vi "Startup_Main.vi"(11 "Message Steps Ref":refnum<vi>) -> (1 "path":path)   [LabVIEW 2016]
doc: "Follow the below steps:\n1) Run the VI\n2) 1st State is \"Wait For Start Acquisition\"\nSelect the \"StartAcquisition\" from States-Enum and Press Send External Trigger button\n3) 2nd State is \"Read Configuration\"\nSelect the \"CheckConfigChanged\" from States-Enum and Press Send External Trigger button\n4) 3rd State is \"Create Channels\"\nThis will Popup a message and automatically goes to next state\n5) 4th State is \"Start Task\"\nThis will Popup a message and automatically goes to next state\n6) 5th State is \"Acquire Data\"\nThe logic will wait here until the \"StopAcq\" or \"Shutdown\" triggers are received\n7) Select the \"StopAcq\" from States-Enum and Press Send External Trigger button\nThis will Popup a message and automatically goes to first state\n\nNote: \nAny state where the logic is waiting, you can Select the \"StopAcq\" from States-Enum and Press Send External Trigger button\n- This will popup a message and automatically goes to first state\nAny state where the logic is waiting, you can Select the \"Shutdown\" from States-Enum and Press Send External Trigger button\n- This will execute the Shutdown state and terminate the program\nBy Manish Soni"
uses:
  Startup_States.ctl
panel:
  out "path 2":path
  out "Paths":T1
  out "String":string
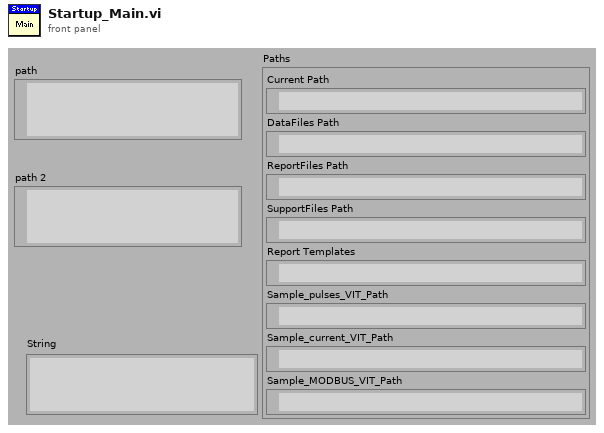
[diagram p1: front panel]
types:
  T1 = cluster{"Current Path":path, "DataFiles Path":path, "ReportFiles Path":path, "SupportFiles Path":path, "Report Templates":path, "Sample_pulses_VIT_Path":path, "Sample_current_VIT_Path":path, "Sample_MODBUS_VIT_Path":path}
  T2 = typedef "Startup_States.ctl" = enum16{"Activation", "Login", "ManageFolderPath", "ReadConfig", "DetectHart485", "ManageLastState", "Close"}
  T3 = enum32{"invalid app kind", "Development System", "Run Time System", "Student Edition", "Embedded LabVIEW", "Evaluation", "Custom"}
  T4 = enum32{"Invalid", "Standard", "Closed", "Hidden", "Minimized", "Maximized"}
  T5 = cluster{"Current Path":path, "DataFiles Path":path, "ReportFiles Path":path, "SupportFiles Path":path, "ReportTemplate Path":path, "Sample_pulses_VIT_Path":path, "Sample_current_VIT_Path":path, "Sample_MODBUS_VIT_Path":path}
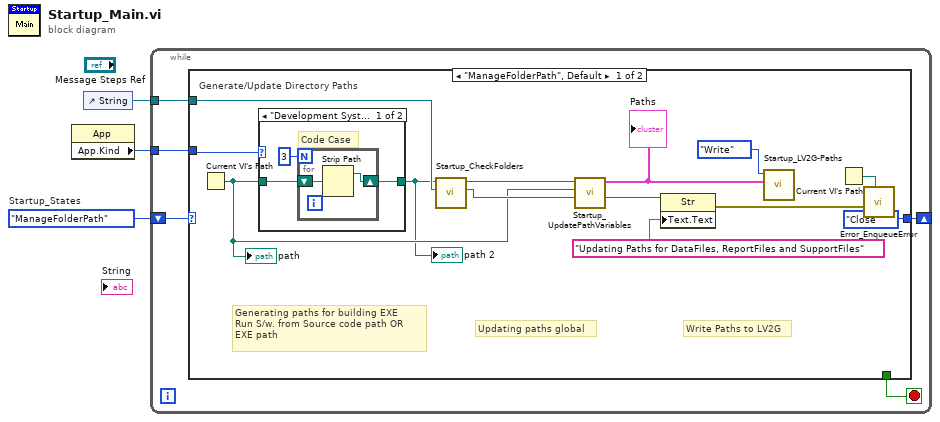
[diagram p0: block diagram]
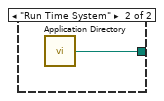
[diagram p2: hidden frame]
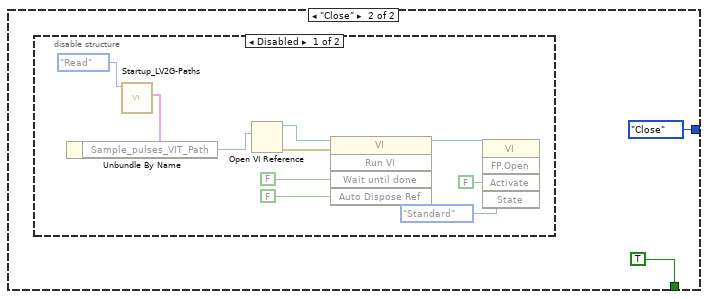
[diagram p3: hidden frame]
diagram:
  w3 = Startup_States."ManageFolderPath"  # Startup_States
  n1 = property class="App"() -> ("App.Kind"=w1:T3)  [unwired: 2 in, 2 out]
  n2 = control-ref of="String"() -> (w2:refnum<vi>)
  n3 = while {
    tunnel: w2 -> [w7]
    shift-right: [w6] -> _
    shift-left: w3 -> [w8]
    tunnel: w1 -> [w4]
    stop <- w5 stop-if-true
    n4 = case shown="\"ManageFolderPath\", Default" w8 {
      tunnel: w7 -> [w13 _]
      tunnel: [Startup_States."Close" ("Startup_States") Startup_States."Close" ("Startup_States")] -> w6
      tunnel: [_ TRUE] -> w5
      tunnel: w4 -> [w10 _]
      frame "ManageFolderPath", Default {
        # "Generate/Update Directory Paths"
        # "Write Paths to LV2G"
        # "Generating paths for building EXE\nRun S/w. from Source code path OR\nEXE path"
        # "Updating paths global"
        n5 = Current VI's Path() -> (path=w11:path)
        "path" <- w11
        n6 = case shown="\"Development System\", Default" w10 {
          tunnel: w11 -> [w24 _]
          tunnel: [w22 w27] -> w9
          frame "Development System", Default {
            # "Code Case"
            n7 = for {
              N: 3 ("f") -> [_]
              shift-right: [w25] -> w22
              shift-left: w24 -> [w26]
              n8 = Strip Path(path=w26) -> (stripped path=w25:path)  [unwired: 1 out]
            }
          }
          frame "Run Time System" {
            n9 = call <vilib>:"Application Directory.vi"() -> ("Application Directory"=w27:path)
          }
        }
        "path 2" <- w9
        n10 = call "Startup_CheckFolders.vi"("Message Steps Ref In"=w13, "MainVIPathIn"=w9) -> ("Message Steps Ref Out"=w17:refnum<vi>, "MainVIPathOut"=w16:path)  [unwired: 2 in, 6 out]
        n11 = call "Startup_UpdatePathVariables.vi"("Message Steps Ref In"=w17, "MainVI Path"=w11, "MainFolder Path"=w16) -> ("Message Steps Ref Out"=w19:refnum<vi>, "Paths"=w15:T5)  [unwired: 1 in, 6 out]
        "Paths" <- w15
        n12 = property class="Str"(reference=w19, "Text.Text"="Updating Paths for DataFiles, ReportFiles and SupportFiles") -> (error out=w21:errorcluster)  [unwired: 1 in, 1 out]
        n13 = call "Startup_LV2G-Paths.vi"("Paths"=w15, "Action"=enum16{"Read", "Write"}."Write") -> ()  [unwired: 2 in, 8 out]
        n14 = Current VI's Path() -> (path=w20:path)
        n15 = call "Error_EnqueueError.vi"("SourcePath"=w20, "Error in"=w21) -> ()  [unwired: 1 in, 9 out]
      }
      frame "Close" {
        n16 = disable-structure shown="Disabled" {
          frame Disabled {
            n17 = call "Startup_LV2G-Paths.vi"("Action"=enum16{"Read", "Write"}."Read") -> ("Paths"=w34:T5)  [unwired: 3 in, 7 out]
            n18 = Unbundle By Name(w34) -> ("Sample_pulses_VIT_Path"=w33:path)
            n19 = Open VI Reference(vi path=w33) -> (vi reference=w36:refnum<vi>, error out=w37:errorcluster)  [unwired: 5 in]
            n20 = invoke class="VI" method="Run VI"(reference=w36, error in=w37, "Wait until done"=FALSE ("Wait Until Done"), "Auto Dispose Ref"=FALSE ("Auto Dispose Reference")) -> (reference out=w32:refnum<vi>)  [unwired: 1 in, 4 out]
            n21 = invoke class="VI" method="FP.Open"(reference=w32, "Activate"=FALSE ("Activate?"), "State"=T4."Standard") -> ()  [unwired: 2 in, 5 out]
          }
          frame Enabled {
          }
        }
      }
    }
  }
